vi "Shooter Bang-Bang Controller.vi"(8 "Right Current RPM":dbl, 9 "Right Target RPM":dbl, 10 "Left Current RPM":dbl, 11 "Left Target RPM":dbl) -> (2 "Right Output Power":dbl, 3 "Left Output Power":dbl)   [LabVIEW 2015]
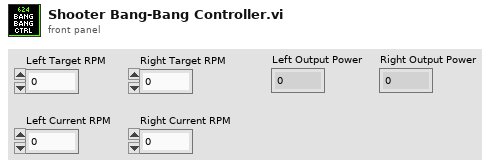
[diagram p1: front panel]
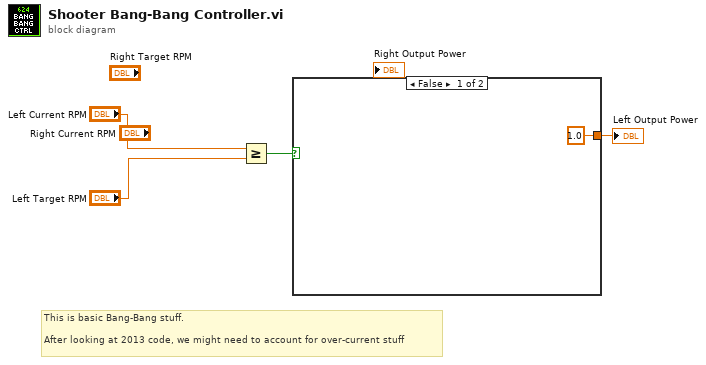
[diagram p0: block diagram]
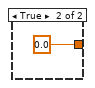
[diagram p2: hidden frame]
diagram:
  # "This is basic Bang-Bang stuff.\n\nAfter looking at 2013 code, we might need to account for over-current stuff"
  n1 = Greater Or Equal?(x="Left Current RPM", y="Left Target RPM") -> (x >= y?=w2:bool)
  n2 = case shown="False" w2 {
    tunnel: [1.0 ("Output Power") 0.0 ("Output Power")] -> w1
    frame False {
    }
    frame True {
    }
  }
  "Left Output Power" <- w1
